vi "RSZVB Global Data.vi"() -> ()   [LabVIEW 2015]
panel:
  in  "Session Data":T1(array[cluster])
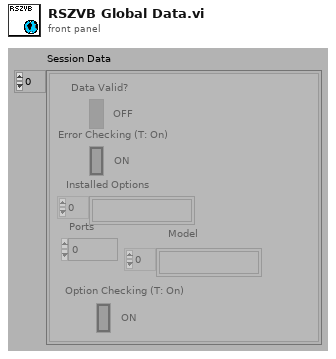
[diagram p1: front panel]
types:
  T1 = cluster{"Error Checking (T: On)":bool, "Installed Options":string[], "Data Valid?":bool, "Ports":i32, "Model":string[], "Option Checking (T: On)":bool}[]
diagram:
